vi "Login_try.rt.vi"() -> ()   [LabVIEW 2012]
uses:
  <vilib>/Utility/miscctls.llb/LVPointTypeDef.ctl
panel:
  in  "User name":u16(ring) items=["a", "ATE"]
  out "Table out":string[][](array[string])=[["Administrator", "Administrator", "ATS"], ["User1", "", ""], ["User2", "", ""]]
  out "Success":bool
  out "loginPath":path
  in  "btnExit":bool
  in  "btnLogin":bool
  in  "Password":string
  in  "User name":string
  # "Ent"
  # "Esc"
  # "Logon Information"
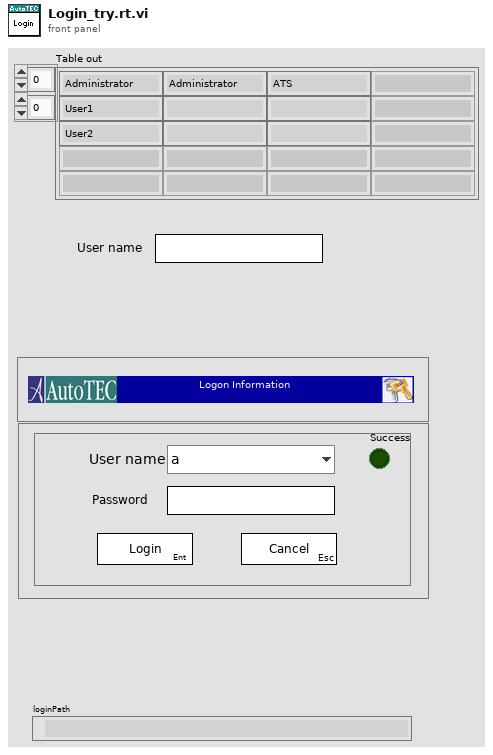
[diagram p1: front panel]
types:
  T1 = typedef "LVPointTypeDef.ctl" = cluster{"Horizontal":i16, "Vertical":i16}
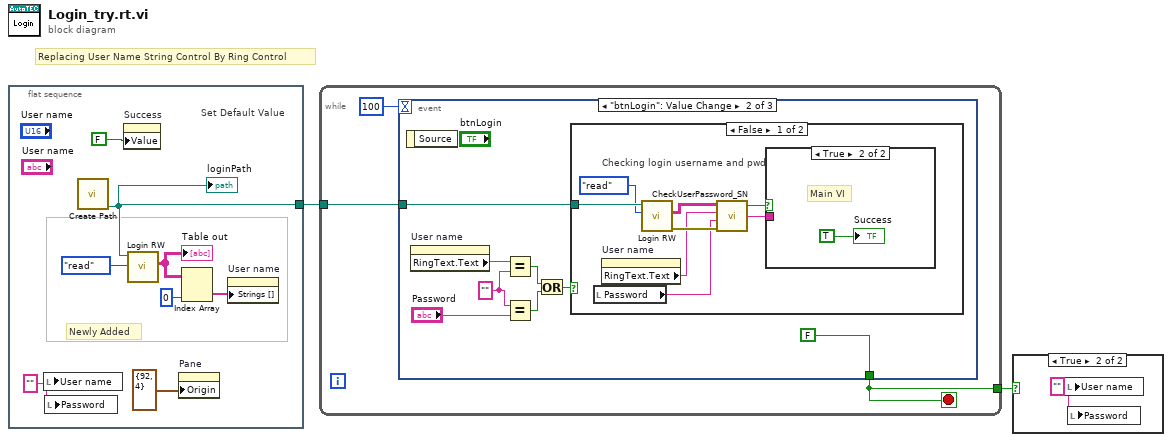
[diagram p0: block diagram]
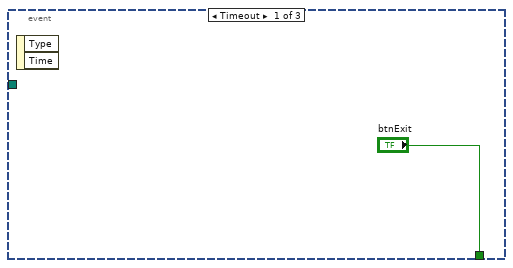
[diagram p3: hidden frame]
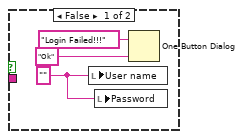
[diagram p4: hidden frame]
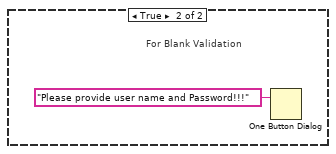
[diagram p5: hidden frame]
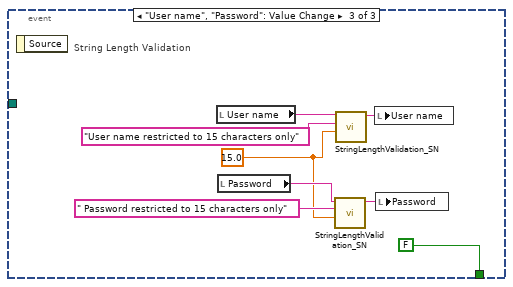
[diagram p6: hidden frame]
diagram:
  # "Replacing User Name String Control By Ring Control"
  n1 = flat-sequence {
    tunnel: [w4] -> w1
    frame #0 {
      w10 = "" ("Password")
      # "Newly Added"
      # "Set Default Value"
      n2 = local write "User name"(w10) -> ()
      n3 = local write "Password"(w10) -> ()
      n4 = call "Create Path.vi"() -> ("Login path"=w4:path)  [unwired: 11 in]
      "loginPath" <- w4
      n5 = property on="Success" class="Bool (strict)"("Value"=FALSE ("Success")) -> ()  [unwired: 2 in, 2 out]
      n6 = call "Login RW.vi"("Enum"=enum16{"write", "read"}."read", "Path in"=w4) -> ("Table out"=w8:string[][])  [unwired: 7 in, 2 out]
      "Table out" <- w8
      n7 = property on="Pane" class="Pane"("Origin"=T1 {"Horizontal"=92, "Vertical"=4} ("Point")) -> ()  [unwired: 2 in, 2 out]
      n8 = Index Array(array=w8, index (col)=0 ("disabled index (col)")) -> (element=w6:string[])  [unwired: 1 in]
      n9 = property on="User name" class="Ring (strict)"("Strings []"=w6) -> ()  [unwired: 2 in, 2 out]
    }
  }
  n10 = while {
    tunnel: [w12] -> w2
    tunnel: w1 -> [w11]
    stop <- w12 stop-if-true
    n11 = event shown="[1] \"btnLogin\": Value Change" {
      selector: _ -> [_ _ _]
      dyn-events: _ -> [_ _ _]
      timeout: 100 -> [_ _ _]
      tunnel: ["btnExit" FALSE ("btnExit") FALSE ("btnExit")] -> w12
      tunnel: w11 -> [_ w16 _]
      event Timeout {
        n12 = event-data() -> ()  [unwired: 1 in, 2 out]
      }
      event "btnLogin": Value Change {
        w18 = "" ("y")
        n13 = event-data() -> ()  [unwired: 1 in, 1 out]
        n14 = property on="User name" class="Ring (strict)"() -> ("RingText.Text"=w15:string)  [unwired: 2 in, 2 out]
        n15 = Equal?(x=w15, y=w18) -> (x = y?=w22:bool)
        n16 = Equal?(x=w18, y="Password") -> (x = y?=w21:bool)
        n17 = Or(x=w22, y=w21) -> (x .or. y?=w20:bool)
        n18 = case shown="False" w20 {
          tunnel: w16 -> [w28 _]
          frame False {
            # "Checking login username and pwd"
            n19 = local read "Password"() -> (w24:string)
            n20 = property on="User name" class="Ring (strict)"() -> ("RingText.Text"=w23:string)  [unwired: 2 in, 2 out]
            n21 = call "Login RW.vi"("Enum"=enum16{"write", "read"}."read", "Path in"=w28) -> ("error out"=w27:errorcluster, "Table out"=w25:string[][])  [unwired: 7 in, 1 out]
            n22 = call "CheckUserPassword_SN.vi"("error in (no error)"=w27, "Password"=w24, "User name"=w23, "Arr_LoginDetails"=w25) -> ("PermissionLevel"=w29:string, "Bool_LoginTrue"=w30:bool)  [unwired: 1 out]
            n23 = case shown="True" w30 {
              tunnel: w29 -> [_ _]
              frame False {
                w31 = "" ("Password")
                n24 = local write "User name"(w31) -> ()
                n25 = local write "Password"(w31) -> ()
                n26 = One Button Dialog(message="Login Failed!!!", button name ("OK")="Ok") -> ()  [unwired: 1 out]
              }
              frame True {
                # "Main VI"
                "Success" <- TRUE ("Boolean")
              }
            }
          }
          frame True {
            # "For Blank Validation"
            n27 = One Button Dialog(message="Please provide user name and Password!!!") -> ()  [unwired: 1 in, 1 out]
          }
        }
      }
      event "User name", "Password": Value Change {
        w38 = 15.0 ("NumbertoRestric")
        # "String Length Validation"
        n28 = event-data() -> ()  [unwired: 1 in, 1 out]
        n29 = local read "User name"() -> (w43:string)
        n30 = local read "Password"() -> (w40:string)
        n31 = call "StringLengthValidation_SN.vi"("NumbertoRestric"=w38, "MessagetoDisplay"=" Password restricted to 15 characters only" ("message"), "StringToValidate"=w40) -> ("StringAfterValidation"=w37:string)  [unwired: 8 in]
        n32 = call "StringLengthValidation_SN.vi"("NumbertoRestric"=w38, "MessagetoDisplay"="User name restricted to 15 characters only" ("message"), "StringToValidate"=w43) -> ("StringAfterValidation"=w41:string)  [unwired: 8 in]
        n33 = local write "User name"(w41) -> ()
        n34 = local write "Password"(w37) -> ()
      }
    }
  }
  n35 = case shown="True" w2 {
    frame False {
    }
    frame True {
      w44 = "" ("User name")
      n36 = local write "User name"(w44) -> ()
      n37 = local write "Password"(w44) -> ()
    }
  }
